vi "Check_Battery.vi"() -> ()   [LabVIEW 2014]
uses:
  <userlib>/UCSD Robotics Lab/Robotics-Cape/LV/libroboticscape.lvlib
panel:
  out "Battery Connection":bool
  out "Timing Block":T1 {"Actual Hz" format="%#_3g"; "Dt" format="%#_4g"; "Average Hz" format="%#_4g"}
  out "Voltage":cluster{"Pack ":sgl, "Jack ":sgl, "Cell ":sgl} {"Cell" format="%#_4g"; "Jack" format="%#_4g"; "Pack" format="%#_4g"}
  out "Iteration counter":i32
  out "State":T2(ring)
  in  "stop":bool
  # "Always stop the VI using the rectangular STOP button above, never with the round stopsign (Abort)"
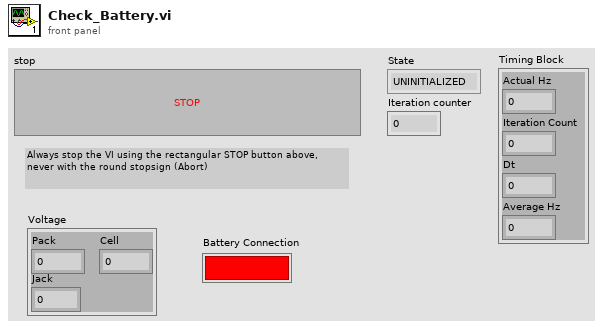
[diagram p1: front panel]
types:
  T1 = cluster{"Actual Hz":dbl, "Iteration Count":dbl, "Dt":dbl, "Average Hz":dbl}
  T2 = enum16{"UNINITIALIZED", "RUNNING", "PAUSED", "EXITING"}
  T3 = enum16{"UNINITIALIZED", "RUNING", "PAUSED", "EXITING"}
  T4 = cluster{"function return":sgl, "function return":sgl, sgl}
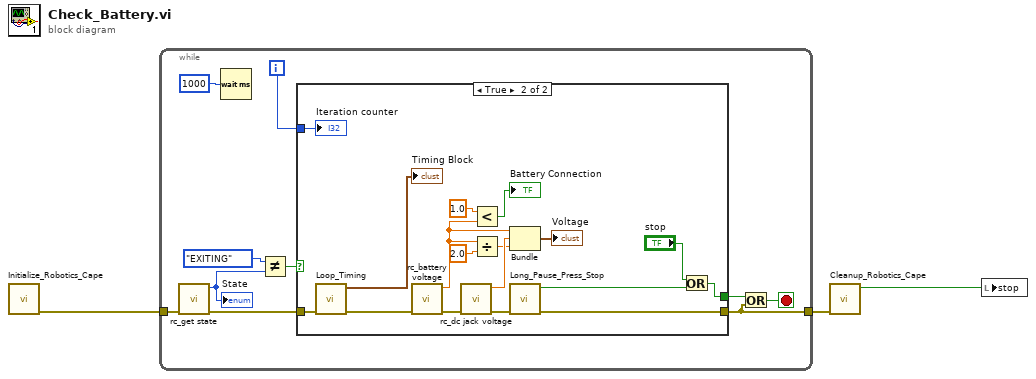
[diagram p0: block diagram]
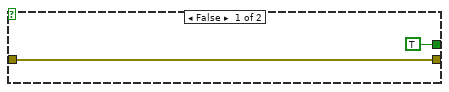
[diagram p2: hidden frame]
diagram:
  n1 = call "Initialize_Robotics_Cape.vi"() -> ("error out"=w3:errorcluster)  [unwired: 11 in]
  n2 = while {
    tunnel: w3 -> [w12]
    tunnel: [w6] -> w2
    i -> [w11]
    stop <- w13 stop-if-true
    n3 = call <userlib>:"rc_get state.vi"("error in (no error)"=w12) -> ("error out"=w7:errorcluster, "function return"=w9:u32)  [unwired: 9 in]
    "State" <- w9
    n4 = Wait (ms)(milliseconds to wait=u32 1000) -> ()  [unwired: 1 out]
    n5 = Not Equal?(x=T3."EXITING" ("State 2"), y=w9) -> (x != y?=w8:bool)
    n6 = case shown="True" w8 {
      tunnel: w11 -> [_ w32]
      tunnel: w7 -> [w15 w25]
      tunnel: [w15 w16] -> w6
      tunnel: [TRUE ("stop") w18] -> w5
      frame False {
      }
      frame True {
        n7 = call "Loop_Timing.vi"("error in"=w25) -> ("error out"=w24:errorcluster, "Timing Block"=→"Timing Block":T1)  [unwired: 9 in]
        n8 = call <userlib>:"rc_battery voltage.vi"("error in (no error)"=w24) -> ("error out"=w31:errorcluster, "function return"=w21:sgl)  [unwired: 9 in]
        n9 = call <userlib>:"rc_dc jack voltage.vi"("error in (no error)"=w31) -> ("error out"=w17:errorcluster, "function return"=w28:sgl)  [unwired: 9 in]
        n10 = Less?(x=sgl 1.0 ("y"), y=w21) -> (x < y?=→"Battery Connection":bool)
        n11 = Divide(x=w21, y=sgl 2.0) -> (x/y=w27:sgl)
        n12 = Bundle("function return"=w21, "function return"=w28, w27) -> (→"Voltage":T4)  [unwired: 1 in]
        n13 = call "Long_Pause_Press_Stop.vi"("error in (no error)"=w17) -> ("error out"=w16:errorcluster, "Stop"=w20:bool)  [unwired: 9 in]
        n14 = Or(x="stop", y=w20) -> (x .or. y?=w18:bool)
        "Iteration counter" <- w32
      }
    }
    n15 = Or(x=w5, y=w6) -> (x .or. y?=w13:bool)
  }
  n16 = call "Cleanup_Robotics_Cape.vi"("error in (no error)"=w2) -> ("Stop Local Variabl"=w1:bool)  [unwired: 9 in, 1 out]
  n17 = local write "stop"(w1) -> ()
